vi "BASE.WriteConfig.vi"(8 "error in (no error)":errorcluster, 11 "BASE.Device in":refnum<class "BASE.Device.lvclass">) -> (0 "error out":errorcluster, 3 "BASE.Device out":refnum<class "BASE.Device.lvclass">)   [LabVIEW 2019, in "BASE.Device.lvlib" / "BASE.Device.lvclass"]
uses:
  BASE.Device.lvclass
  Subsystems/BASE/BASE/BASE.lvclass
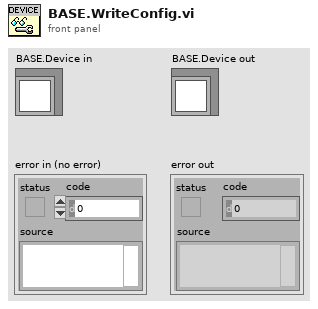
[diagram p1: front panel]
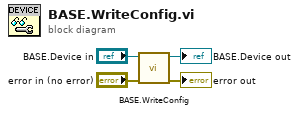
[diagram p0: block diagram]
diagram:
  n1 = call-parent "BASE.WriteConfig.vi"("error in (no error)"="error in (no error)", "BASE in"="BASE.Device in") -> ("error out"=→"error out":errorcluster, "BASE out"=→"BASE.Device out":refnum<class "BASE.Device.lvclass">)  [unwired: 8 in]
